vi "filter sampled data.vi"(7 "low cutoff freq: fl":dbl=30.0 format="%0.4f", 9 "last data set":cluster{"t":dbl[], "x":dbl[]}, 10 "t x data":cluster{"t":dbl[], "x":dbl[]}) -> (1 "current data set":cluster{"t":dbl[], "x":dbl[]}, 2 "t x data filetered":cluster{"t":dbl[], "x":dbl[]})   [LabVIEW 2010]
uses:
  <vilib>/Analysis/3filter.llb/Filter Passband Type.ctl
  <vilib>/Analysis/3filter.llb/Bessel Filter (DBL).vi
  <vilib>/gmath/NI_Gmath.lvlib
  <vilib>/Analysis/NI_AALBase.lvlib
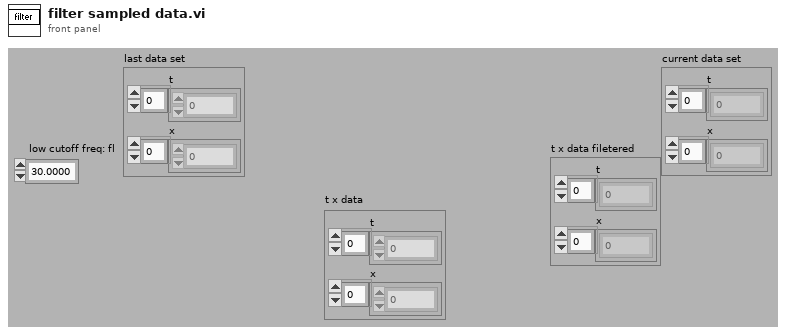
[diagram p1: front panel]
types:
  T1 = typedef "NI_AALBase.lvlib/Filter Passband Type.ctl" = enum32{"Lowpass", "Highpass", "Bandpass", "Bandstop"}
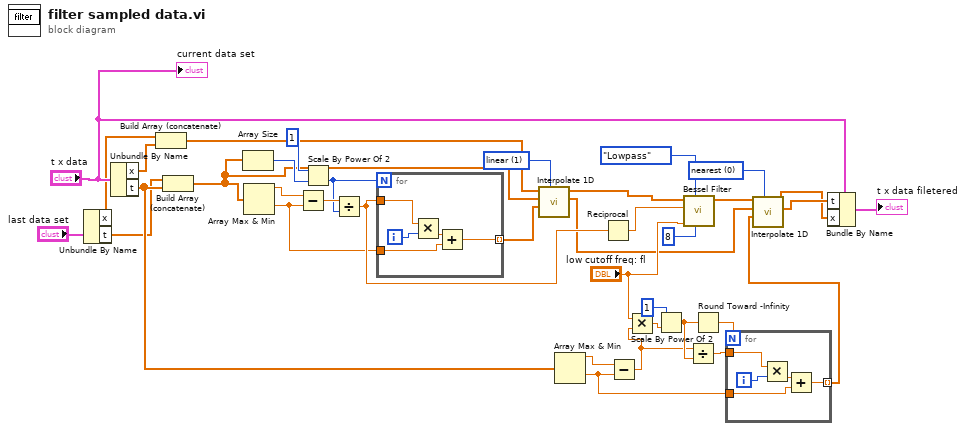
[diagram p0: block diagram]
diagram:
  w14 = 0 items=["nearest", "linear", "spline", "cubic Hermite", "Lagrange"] ("method")
  w35 = 1 items=["nearest", "linear", "spline", "cubic Hermite", "Lagrange"] ("method")
  n1 = Unbundle By Name("last data set") -> ("x"=w2:dbl[], "t"=w1:dbl[])
  n2 = Unbundle By Name("t x data") -> ("x"=w6:dbl[], "t"=w7:dbl[])
  n3 = Build Array (concatenate)(w2, w6) -> (w5:dbl[])
  n4 = Build Array (concatenate)(w1, w7) -> (w4:dbl[])
  n5 = Array Size(array=w4) -> (size(s)=w17:i32)
  n6 = Array Max & Min(array=w4) -> (max value=w37:dbl, min value=w26:dbl)  [unwired: 2 out]
  n7 = Subtract(x=w37, y=w26) -> (x-y=w23:dbl)
  n8 = Scale By Power Of 2(n=1, x=w17) -> (x*2^n=w18:i32)
  n9 = Divide(x=w23, y=w18) -> (x/y=w30:dbl)
  n10 = for {
    N: w18 -> [_]
    tunnel: w30 -> [w41]
    tunnel: w26 -> [w39]
    tunnel: [w38] -> w36 mode=indexing
    i -> [w42]
    n11 = Multiply(x=w41, y=w42) -> (x*y=w40:dbl)
    n12 = Add(x=w40, y=w39) -> (x+y=w38:dbl)
  }
  n13 = call <vilib>:"Interpolate 1D.vi"("method"=w35, "xi"=w36, "X"=w4, "Y"=w5) -> ("xi used"=w8:dbl[], "yi"=w9:dbl[])  [unwired: 5 in, 1 out]
  n14 = Array Max & Min(array=w7) -> (max value=w13:dbl, min value=w11:dbl)  [unwired: 2 out]
  n15 = Reciprocal(x=w30) -> (1/x=w32:dbl)
  n16 = Subtract(x=w13, y=w11) -> (x-y=w12:dbl)
  n17 = Multiply(x="low cutoff freq: fl", y=w12) -> (x*y=w28:dbl)
  n18 = Scale By Power Of 2(n=1, x=w28) -> (x*2^n=w24:dbl)
  n19 = call-poly <vilib>:"Bessel Filter.vi"("order"=8, "filter type"=Filter_Passband_Type."Lowpass", "low cutoff freq: fl"="low cutoff freq: fl", "sampling freq: fs"=w32, "X"=w9) -> ("Filtered X"=w31:dbl[])  [unwired: 3 in, 1 out]
  n20 = Divide(x=w12, y=w24) -> (x/y=w25:dbl)
  n21 = Round Toward -Infinity(1:w24) -> (0:w15:dbl)
  n22 = for {
    N: w15 -> [_]
    tunnel: w25 -> [w46]
    tunnel: w11 -> [w44]
    tunnel: [w43] -> w22 mode=indexing
    i -> [w47]
    n23 = Multiply(x=w46, y=w47) -> (x*y=w45:dbl)
    n24 = Add(x=w45, y=w44) -> (x+y=w43:dbl)
  }
  n25 = call <vilib>:"Interpolate 1D.vi"("method"=w14, "xi"=w22, "X"=w8, "Y"=w31) -> ("xi used"=w21:dbl[], "yi"=w20:dbl[])  [unwired: 5 in, 1 out]
  n26 = Bundle By Name(cluster="t x data", "t"=w21, "x"=w20) -> (→"t x data filetered":cluster{"t":dbl[], "x":dbl[]})
  "current data set" <- "t x data"
